vi "Modify_Metadata_Channels.vi"(4 "Ch Description Array":T1[](array[typedef]) {"Duty" format="%016b"; "D" format="%#_5g"; "C" format="%#_5g"; "B" format="%#_5g"; "A" format="%#_5g"}) -> (1 "Ch Description Array Out":T1[](array[typedef]) {"Duty" format="%016b"; "D" format="%#_5g"; "C" format="%#_5g"; "B" format="%#_5g"; "A" format="%#_5g"})   [LabVIEW 2018]
uses:
  ADAM Controls/Ch_description_ADAM.ctl
  ADAM Controls/Module_type_ADAM.ctl
  ADAM Controls/Function_ADAM.ctl
  ADAM Controls/Channel_State.ctl
  ADAM Controls/Calib_type_ADAM.ctl
  ADAM Controls/Address.ctl
  Anemometry/Anemometry Sub Vis/Globals/Preference_global.vi
panel:
  in  "Cluster Template":cluster{"Channel Name":string, "Menu Ring":bool}
  in  "Channel Types":T7(array[cluster])
  in  "Select Channels to Activate":i32[](listbox)
  in  "Add a New Channel":bool
  in  "stop":bool
  in  "OK":bool
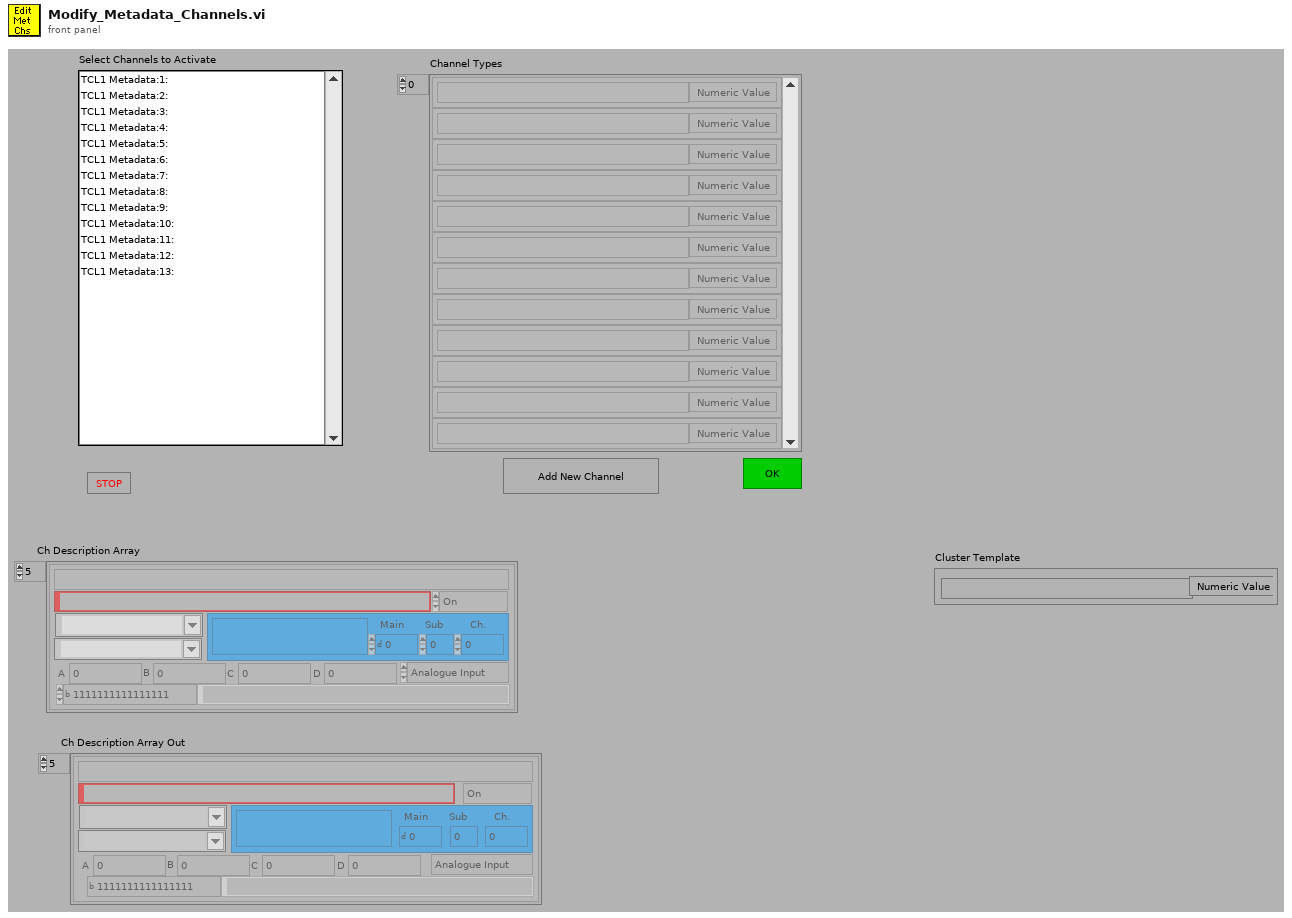
[diagram p1: front panel]
types:
  T1 = typedef "Ch_description_ADAM.ctl" = cluster{"Ch Name":string, "Type":T2, "Function":T3, "Ch State":T4, "Calibration type":T5, "A":dbl, "B":dbl, "C":dbl, "D":dbl, "Comments":string, "Address":T6, "String":string, "Duty":u16}
  T2 = typedef "Module_type_ADAM.ctl" = string
  T3 = typedef "Function_ADAM.ctl" = enum16{"Analogue Input", "Digital Input", "Event counter", "Event rate", "Analogue Output", "Digital Output", "Relay Output"}
  T4 = typedef "Channel_State.ctl" = enum16{"On", "Off", "Always On", "Always Off"}
  T5 = typedef "Calib_type_ADAM.ctl" = string
  T6 = typedef "Address.ctl" = cluster{"Main":i32, "Ch.":i32, "Sub":i32, "Port Name":string}
  T7 = cluster{"Channel Name":string, "Menu Ring":bool}[]
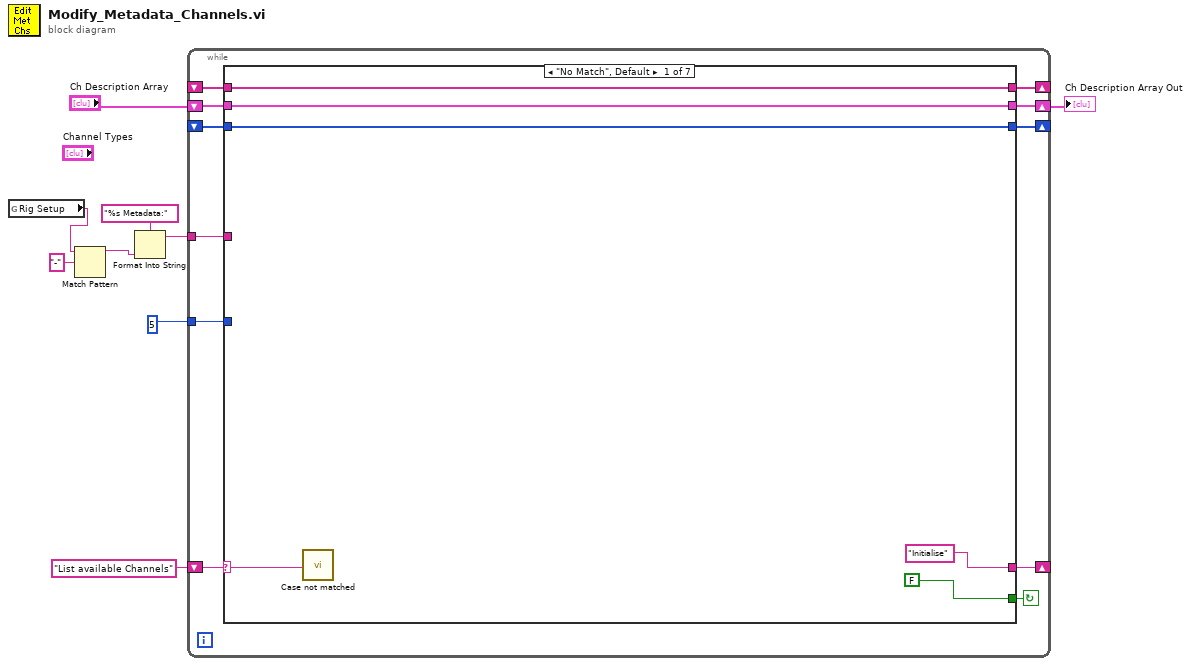
[diagram p0: block diagram]
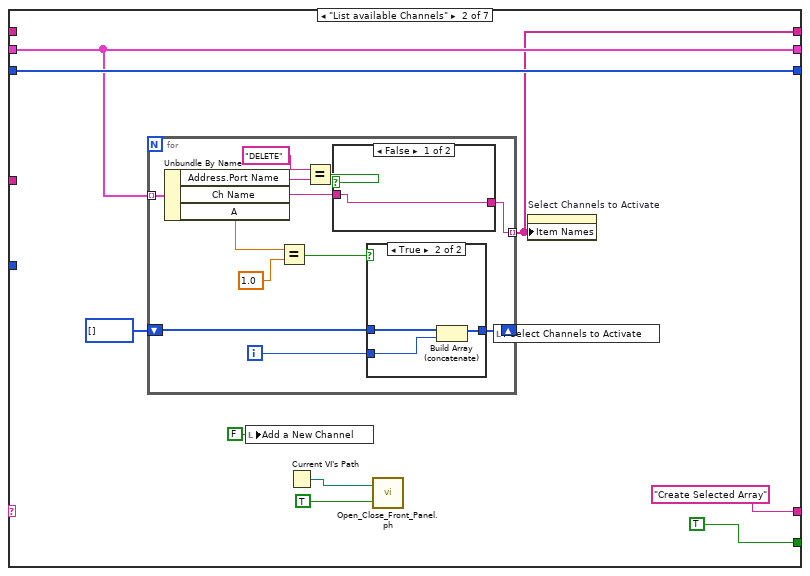
[diagram p2: hidden frame]
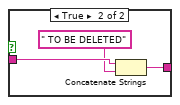
[diagram p3: hidden frame]
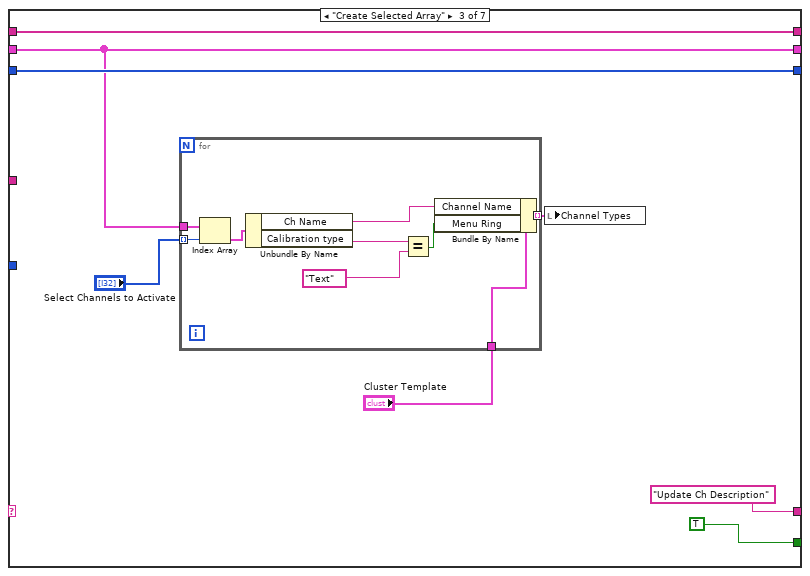
[diagram p5: hidden frame]
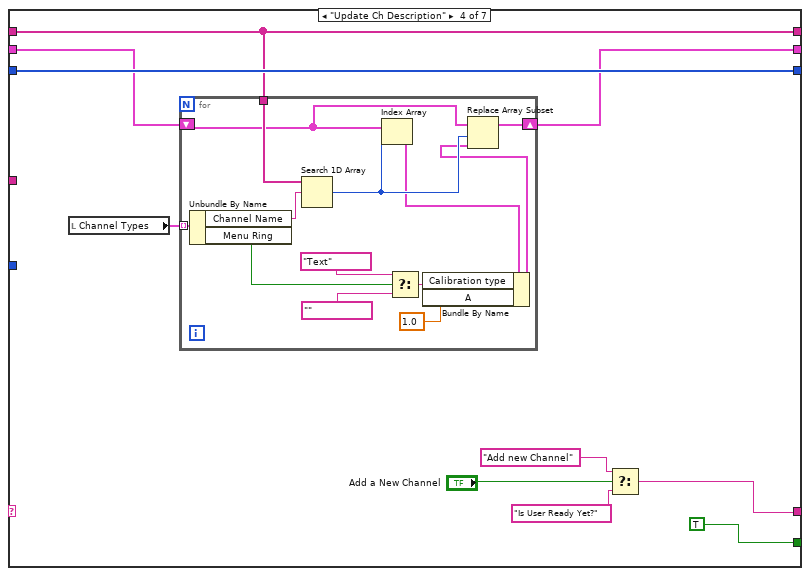
[diagram p6: hidden frame]
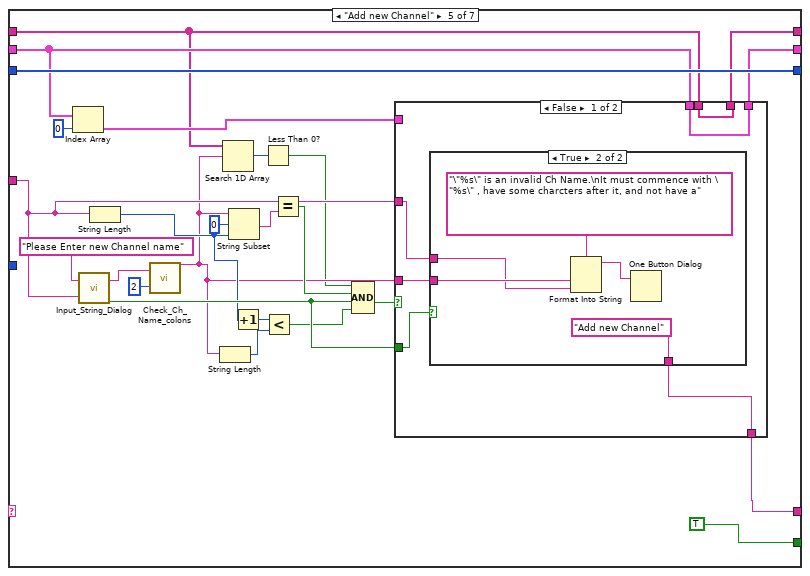
[diagram p7: hidden frame]
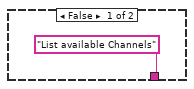
[diagram p8: hidden frame]
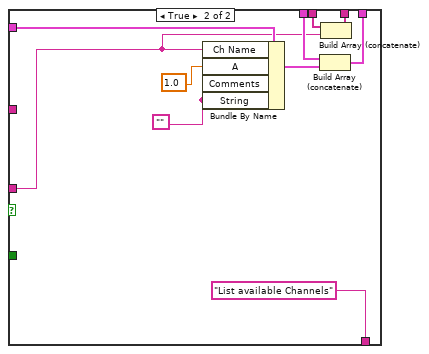
[diagram p9: hidden frame]
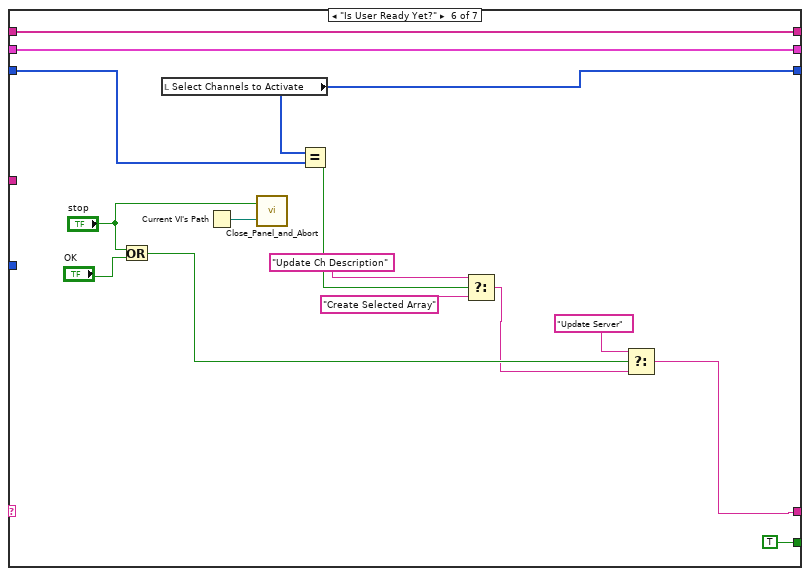
[diagram p10: hidden frame]
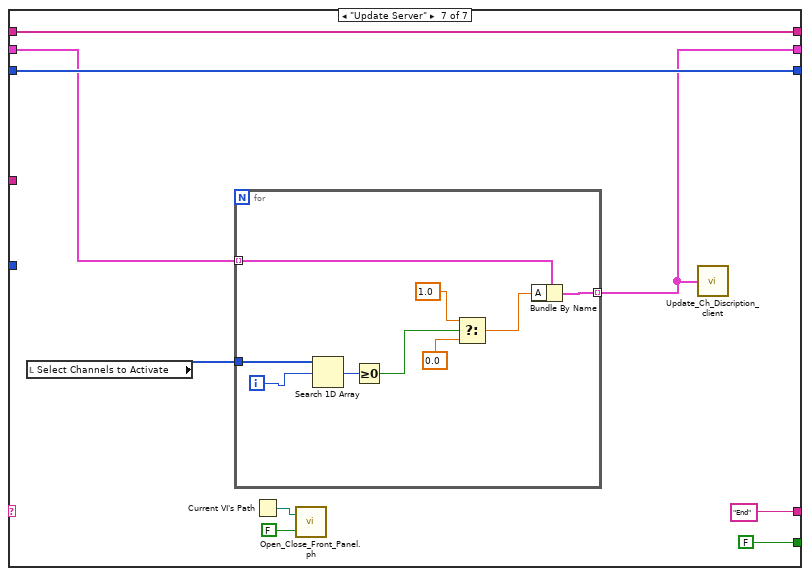
[diagram p11: hidden frame]
diagram:
  n1 = global read "Preference_global.vi" "Rig Setup"() -> (w2:string)
  n2 = Match Pattern(string=w2, regular expression="-") -> (before substring=w1:string)  [unwired: 4 out]
  n3 = Format Into String(format string="%s Metadata:" ("Format String"), w1) -> (resulting string=w7:string)  [unwired: 2 in, 1 out]
  n4 = while {
    tunnel: 5 -> [w10]
    tunnel: w7 -> [w11]
    shift-left: _ -> [w14]
    shift-right: [w13] -> _
    shift-left: _ -> [w15]
    shift-right: [w17] -> _
    shift-left: "Ch Description Array" -> [w16]
    shift-right: [w18] -> w4
    shift-left: "List available Channels" -> [w19]
    shift-right: [w12] -> _
    stop <- w20 continue-if-true
    n5 = case shown="\"No Match\", Default" w19 {
      selector: w19 -> [w21 _ _ _ _ _ _]
      tunnel: [FALSE TRUE TRUE TRUE TRUE TRUE ("T button?") FALSE ("T button?")] -> w20
      tunnel: ["Initialise" "Create Selected Array" "Update Ch Description" w74 w108 w144 "End"] -> w12
      tunnel: [w24 w33 w60 w80 w116 w158 w161] -> w18
      tunnel: [w23 w34 w62 w82 w120 w152 w164] -> w17
      tunnel: w16 -> [w24 w33 w60 w79 w115 w158 w163]
      tunnel: w15 -> [w23 w34 w62 w82 w120 w151 w164]
      tunnel: w14 -> [w22 _ w57 w78 w100 w153 w165]
      tunnel: [w22 w30 w57 w78 w114 w153 w165] -> w13
      tunnel: w11 -> [_ _ _ _ w109 _ _]
      tunnel: w10 -> [_ _ _ _ _ _ _]
      frame "No Match", Default {
        n6 = call "Case not matched.vi"("Case Name not Matched"=w21) -> ()
      }
      frame "List available Channels" {
        n7 = for {
          tunnel: w33 -> [w48] mode=indexing
          tunnel: [w37] -> w30 mode=indexing
          shift-right: [w43] -> w31
          shift-left: i32[] [] -> [w44]
          i -> [w42]
          n8 = Unbundle By Name(w48) -> ("Address.Port Name"=w41:string, "Ch Name"=w38:string, "A"=w47:dbl)
          n9 = Equal?(x=w47, y=1.0) -> (x = y?=w45:bool)
          n10 = Equal?(x="DELETE", y=w41) -> (x = y?=w39:bool)
          n11 = case shown="False" w39 {
            tunnel: w38 -> [w49 w52]
            tunnel: [w49 w50] -> w37
            frame False {
            }
            frame True {
              n12 = Concatenate Strings(w52, " TO BE DELETED" ("string")) -> (w50:string)
            }
          }
          n13 = case shown="True" w45 {
            tunnel: w44 -> [w53 w56]
            tunnel: [w53 w55] -> w43
            tunnel: w42 -> [_ w54]
            frame False {
            }
            frame True {
              n14 = Build Array (concatenate)(w56, w54) -> (w55:i32[])
            }
          }
        }
        n15 = local write "Add a New Channel"(FALSE ("Add a New Channel")) -> ()
        n16 = Current VI's Path() -> (path=w28:path)
        n17 = call "Open_Close_Front_Panel.ph.vi"("Front Panel Window:Open"=TRUE, "VI path"=w28) -> ()  [unwired: 2 out]
        n18 = local write "Select Channels to Activate"(w31) -> ()
        n19 = property on="Select Channels to Activate" class="LstBox (strict)"("Item Names"=w30) -> ()  [unwired: 2 in, 2 out]
      }
      frame "Create Selected Array" {
        n20 = for {
          tunnel: "Select Channels to Activate" -> [w73] mode=indexing
          tunnel: w60 -> [w72]
          tunnel: "Cluster Template" -> [w68]
          tunnel: [w65] -> w58 mode=indexing
          n21 = Index Array(array=w72, index=w73) -> (element=w71:T1)
          n22 = Unbundle By Name(w71) -> ("Ch Name"=w66:string, "Calibration type"=w70:T5)
          n23 = Equal?(x=w70, y=T5 "Text" ("Calibration Type")) -> (x = y?=w67:bool)
          n24 = Bundle By Name(cluster=w68, "Channel Name"=w66, "Menu Ring"=w67) -> (w65:cluster{"Channel Name":string, "Menu Ring":bool})
        }
        n25 = local write "Channel Types"(w58) -> ()
      }
      frame "Update Ch Description" {
        n26 = local read "Channel Types"() -> (w81:T7)
        n27 = for {
          tunnel: w81 -> [w96] mode=indexing
          tunnel: w78 -> [w95]
          shift-right: [w88] -> w80
          shift-left: w79 -> [w89]
          n28 = Unbundle By Name(w96) -> ("Channel Name"=w94:string, "Menu Ring"=w93:bool)
          n29 = Search 1D Array(1D array=w95, element=w94) -> (index of element=w90:i32)  [unwired: 1 out]
          n30 = Index Array(array=w89, index=w90) -> (element=w87:T1)
          n31 = Select(t=T5 "Text" ("Calibration Type"), s=w93, f=T5 "" ("Calibration Type")) -> (s? t:f=w86:T5)
          n32 = Bundle By Name(cluster=w87, "Calibration type"=w86, "A"=1.0 ("Bundle Element")) -> (w84:T1)
          n33 = Replace Array Subset(array=w89, new element=w84, index=w90) -> (w88:T1[])
        }
        n34 = Select(t="Add new Channel", s="Add a New Channel", f="Is User Ready Yet?") -> (s? t:f=w74:string)
      }
      frame "Add new Channel" {
        n35 = Index Array(array=w115, index=0 ("Index")) -> (element=w118:T1)
        n36 = call "Input_String_Dialog.vi"("Value"=w109, "Message to user"="Please Enter new Channel name") -> ("Ok Out"=w107:bool, "Output string"=w106:string)
        n37 = String Length(string=w109) -> (length=w103:i32)
        n38 = call "Check_Ch_Name_colons.vi"("No of Colons"=2, "Ch Name in"=w106) -> ("Ch Name out"=w99:string)
        n39 = String Length(string=w99) -> (length=w104:i32)
        n40 = Search 1D Array(1D array=w100, element=w99) -> (index of element=w98:i32)  [unwired: 1 out]
        n41 = String Subset(string=w99, offset (0)=0, length (rest)=w103) -> (substring=w112:string)
        n42 = Increment(x=w103) -> (x+1=w102:i32)
        n43 = Less Than 0?(x=w98) -> (x < 0?=w97:bool)
        n44 = Less?(x=w102, y=w104) -> (x < y?=w101:bool)
        n45 = Equal?(x=w109, y=w112) -> (x = y?=w111:bool)
        n46 = Compound Arithmetic op=AND(w97, w111, w107, w101) -> (w110:bool)
        n47 = case shown="False" w110 {
          tunnel: w99 -> [w125 w137]
          tunnel: w118 -> [_ w143]
          tunnel: w115 -> [w127 w141]
          tunnel: [w127 w140] -> w116
          tunnel: w100 -> [w126 w139]
          tunnel: [w126 w138] -> w114
          tunnel: w109 -> [w124 _]
          tunnel: [w122 "List available Channels"] -> w108
          tunnel: w107 -> [w123 _]
          frame False {
            n48 = case shown="True" w123 {
              tunnel: w125 -> [_ w133]
              tunnel: w124 -> [_ w131]
              tunnel: ["List available Channels" "Add new Channel"] -> w122
              frame False {
              }
              frame True {
                n49 = Format Into String(format string="\"%s\" is an invalid Ch Name.\nIt must commence with \"%s\" , have some charcters after it, and not have a" ("Format String"), w133, w131) -> (resulting string=w130:string)  [unwired: 2 in, 1 out]
                n50 = One Button Dialog(message=w130) -> ()  [unwired: 2 out]
              }
            }
          }
          frame True {
            w134 = ""
            n51 = Bundle By Name(cluster=w143, "Ch Name"=w137, "A"=1.0 ("Bundle Element"), "Comments"=w134, "String"=w134) -> (w142:T1)
            n52 = Build Array (concatenate)(w141, w142) -> (w140:T1[])
            n53 = Build Array (concatenate)(w139, w137) -> (w138:string[])
          }
        }
      }
      frame "Is User Ready Yet?" {
        n54 = Or(x="stop", y="OK") -> (x .or. y?=w147:bool)
        n55 = local read "Select Channels to Activate"() -> (w152:i32[])
        n56 = Current VI's Path() -> (path=w157:path)
        n57 = call "Close_Panel_and_Abort.vi"("Vi path"=w157, "stop"="stop") -> ()  [unwired: 1 out]
        n58 = Equal?(x=w152, y=w151) -> (x = y?=w149:bool)
        n59 = Select(t="Update Ch Description", s=w149, f="Create Selected Array") -> (s? t:f=w146:string)
        n60 = Select(t="Update Server", s=w147, f=w146) -> (s? t:f=w144:string)
      }
      frame "Update Server" {
        n61 = local read "Select Channels to Activate"() -> (w162:i32[])
        n62 = for {
          tunnel: w163 -> [w174] mode=indexing
          tunnel: w162 -> [w176]
          tunnel: [w173] -> w161 mode=indexing
          i -> [w175]
          n63 = Search 1D Array(1D array=w176, element=w175) -> (index of element=w172:i32)  [unwired: 1 out]
          n64 = Greater Or Equal To 0?(x=w172) -> (x >= 0?=w171:bool)
          n65 = Select(t=1.0, s=w171, f=0.0 ("Bundle Element")) -> (s? t:f=w168:dbl)
          n66 = Bundle By Name(cluster=w174, "A"=w168) -> (w173:T1)
        }
        n67 = Current VI's Path() -> (path=w160:path)
        n68 = call "Open_Close_Front_Panel.ph.vi"("Front Panel Window:Open"=FALSE, "VI path"=w160) -> ()  [unwired: 2 out]
        n69 = call "Update_Ch_Discription_client.vi"("Channels to update In"=w161) -> ()  [unwired: 1 out]
      }
    }
  }
  "Ch Description Array Out" <- w4
